vi "Logging Init.vi"(8 "error in (no error)":errorcluster, 11 "Drive Metrics":T1) -> (0 "error out":errorcluster, 2 "Logging Reference":refnum<file>, 3 "Logging FIFO":refnum<k33>)   [LabVIEW 2015]
uses:
  Drive Train/Drive Metrics.ctl
  Drive Train/Drive States.ctl
  Drive Train/Copilot States.ctl
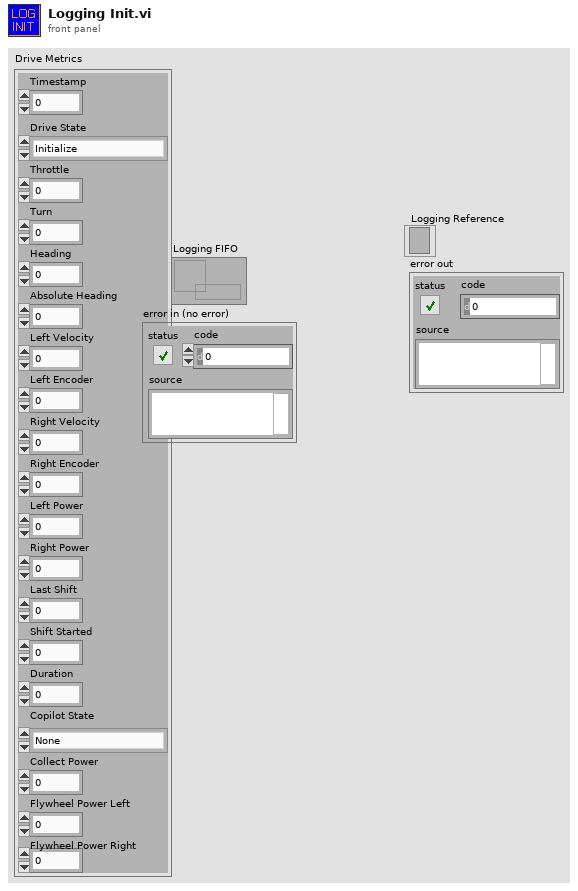
[diagram p1: front panel]
types:
  T1 = typedef "Drive Metrics.ctl" = cluster{"Timestamp":u32, "Drive State":T2, "Throttle":dbl, "Turn":dbl, "Heading":dbl, "Absolute Heading":dbl, "Left Velocity":dbl, "Left Encoder":dbl, "Right Velocity":dbl, "Right Encoder":dbl, "Left Power":dbl, "Right Power":dbl, "Last Shift":u32, "Shift Started":u32, "Duration":i64, "Copilot State":T3, "Collect Power":dbl, "Flywheel Power Left":dbl, "Flywheel Power Right":dbl}
  T2 = typedef "Drive States.ctl" = enum16{"Initialize", "Low Gear", "Up Shift Begin", "Up Shifting", "Up Shift Delay", "High Gear", "Down Shift Begin", "Down Shifting", "Down Shift Delay"}
  T3 = typedef "Copilot States.ctl" = enum16{"None", "Collect", "Eject"}
  T4 = enum16{"open", "replace", "create", "open or create", "replace or create", "replace or create with confirmation"}
  T5 = cluster{"read mode":enum16{"polling", "blocking"}, "write mode":enum16{"polling", "blocking"}}
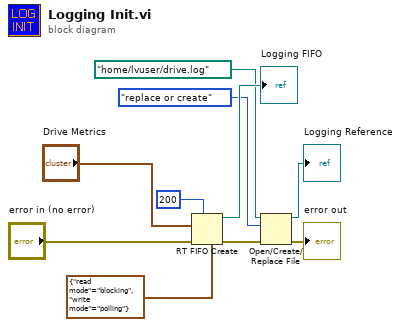
[diagram p0: block diagram]
diagram:
  n1 = RT FIFO Create(1:"Drive Metrics", 3:"error in (no error)", 4:u32 200 ("size (10)"), 7:T5 {"read mode"=enum."blocking", "write mode"=enum."polling"} ("r/w modes (polling,polling)")) -> (8:→"Logging FIFO":refnum<k33>, 11:w2:errorcluster)  [unwired: 4 in, 1 out]
  n2 = Open/Create/Replace File(file path (use dialog)=path "/home/lvuser/drive.log", error in=w2, operation (0:open)=T4."replace or create") -> (refnum out=→"Logging Reference":refnum<file>, error out=→"error out":errorcluster)  [unwired: 3 in, 1 out]
